vi "FdxCmdRxEDEControlCvi.vi"(8 "error in":errorcluster, 9 "EdeControl":T1={"VerificationMode"=enum."FDX_RX_EDE_CHECK_ENA_DEFAULT", "EnableMode"=enum."FDX_RX_EDE_INVDEFAULT", "AgeMax"=0, "MaxSkew"=0, "EdeSnValidWindow"=0}, 10 "UdpControl":T2={"UdpHandle"=0, "NetSelect"=3, "InterruptControl"=enum."FDX_RX_UDP_NOINT"} {"NetSelect" items=["FDX_RX_UDP_ONLY_A"=1, "FDX_RX_UDP_ONLY_B"=2, "FDX_RX_UDP_BOTH"=3]}, 11 "InstrumentHandle":u32) -> (0 "error out":errorcluster, 3 "InstrumentHandle":u32)   [LabVIEW 2020, in "AIM664LV.lvlib"]
doc: "This function allows the user to configure several settings of a EDE Receive Port."
uses:
  AIM664LV.lvlib
  AFDX_LibraryAdmin/FdxGlobalDllPath.vi
panel:
  # "*"
  # "*"
  # "* Note: any logical combination\nof flag can be used."
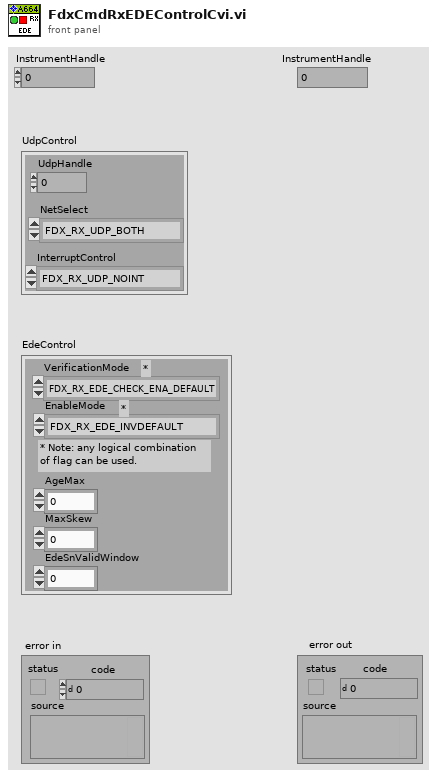
[diagram p1: front panel]
types:
  T1 = cluster{"VerificationMode":enum32{"FDX_RX_EDECHECK_DISA", "FDX_RX_EDE_CHECK_CRCX", "FDX_RX_EDE_CHECK_CRCY", "FDX_RX_EDE_CHECK_ENA_DEFAULT", "FDX_RX_EDE_CHECK_AGE", "UNDEFINED_MODE_1", "UNDEFINED_MODE_2", "UNDEFINED_MODE_3", "FDX_RX_EDE_CHECK_SNINTEG", "UNDEFINED_MODE_4", "FDX_RX_EDE_CHECK_REDMAN"}, "EnableMode":enum32{"FDX_RX_EDE_INVDISCARD", "FDX_RX_EDE_INVCRCX", "FDX_RX_EDE_INVCRCY", "UNDEFINED_MODE_1", "FDX_RX_EDE_INVAGE", "UNDEFINED_MODE_2", "UNDEFINED_MODE_3", "UNDEFINED_MODE_4", "FDX_RX_EDE_INVSN", "UNDEFINED_MODE_5", "UNDEFINED_MODE_6", "UNDEFINED_MODE_7", "UNDEFINED_MODE_8", "UNDEFINED_MODE_9", "UNDEFINED_MODE_10", "FDX_RX_EDE_INVDEFAULT"}, "AgeMax":u32, "MaxSkew":u32, "EdeSnValidWindow":u32}
  T2 = cluster{"UdpHandle":u32, "NetSelect":u32, "InterruptControl":enum32{"FDX_RX_UDP_NOINT", "FDX_RX_UDP_INT", "FDX_RX_UDP_UDF"}}
  T3 = enum32{"FDX_RX_UDP_NOINT", "FDX_RX_UDP_INT", "FDX_RX_UDP_UDF"}
  T4 = enum32{"FDX_RX_EDECHECK_DISA", "FDX_RX_EDE_CHECK_CRCX", "FDX_RX_EDE_CHECK_CRCY", "FDX_RX_EDE_CHECK_ENA_DEFAULT", "FDX_RX_EDE_CHECK_AGE", "UNDEFINED_MODE_1", "UNDEFINED_MODE_2", "UNDEFINED_MODE_3", "FDX_RX_EDE_CHECK_SNINTEG", "UNDEFINED_MODE_4", "FDX_RX_EDE_CHECK_REDMAN"}
  T5 = enum32{"FDX_RX_EDE_INVDISCARD", "FDX_RX_EDE_INVCRCX", "FDX_RX_EDE_INVCRCY", "UNDEFINED_MODE_1", "FDX_RX_EDE_INVAGE", "UNDEFINED_MODE_2", "UNDEFINED_MODE_3", "UNDEFINED_MODE_4", "FDX_RX_EDE_INVSN", "UNDEFINED_MODE_5", "UNDEFINED_MODE_6", "UNDEFINED_MODE_7", "UNDEFINED_MODE_8", "UNDEFINED_MODE_9", "UNDEFINED_MODE_10", "FDX_RX_EDE_INVDEFAULT"}
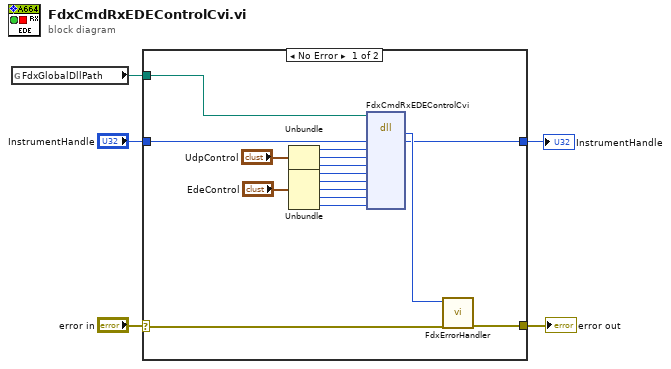
[diagram p0: block diagram]
diagram:
  n1 = global read "FdxGlobalDllPath.vi" "FdxGlobalDllPath"() -> (w3:path)
  n2 = case shown="No Error" "error in" {
    selector: "error in" -> [w20 w23]
    tunnel: [w21 w23] -> w5
    tunnel: w3 -> [w8 _]
    tunnel: "InstrumentHandle" -> [w7 w22]
    tunnel: [w6 w22] -> w1
    frame No Error {
      n3 = Unbundle("UdpControl") -> ("UdpHandle"=w17:u32, "NetSelect"=w16:u32, "InterruptControl"=w15:T3)
      n4 = Unbundle("EdeControl") -> ("VerificationMode"=w13:T4, "EnableMode"=w12:T5, "AgeMax"=w11:u32, "MaxSkew"=w10:u32, "EdeSnValidWindow"=w9:u32)
      n5 = dll-call lib="aim_fdx.19.dll" fn="FdxCmdRxEDEControlCvi"(path in=w8, "InstrumentHandle"=w7, "UdpHandle"=w17, "NetSelect"=w16, "InterrupControl"=w15, "VerificationMode"=w13, "EnableMode"=w12, "AgeMax"=w11, "MaxSkew"=w10, "EdeSnValidWindow"=w9) -> ("status"=w19:i32, "InstrumentHandle"=w6:u32)  [unwired: 7 in, 5 out]
      n6 = call "FdxErrorHandler.vi"("error in"=w20, "AIM Error"=w19) -> ("error out"=w21:errorcluster)  [unwired: 9 in]
    }
    frame Error {
    }
  }
  "error out" <- w5
  "InstrumentHandle" <- w1
